vi "parse_to_rio.vi"(4 "error in":errorcluster, 7 "msg in":string) -> (0 "error out":errorcluster, 2 "to_rio":cluster{"set_speed":dbl, "set_steering":dbl}, 3 "msg out":string)   [LabVIEW 2016]
uses:
  <userlib>/ROS for LabVIEW Software/ROS/MessageParsing/std_msgs/subs/parse_float64_scalar.vi
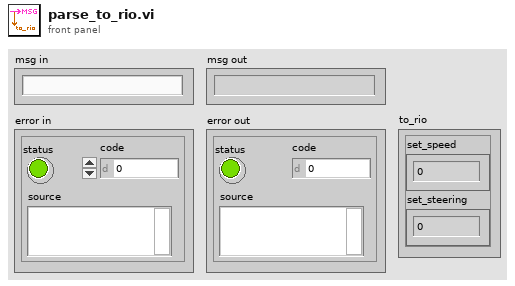
[diagram p1: front panel]
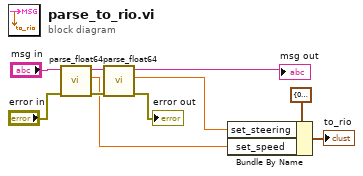
[diagram p0: block diagram]
diagram:
  n1 = call-poly <userlib>:"parse_float64.vi"("error in"="error in", "msg in"="msg in") -> ("error out"=w4:errorcluster, "number"=w1:dbl, "msg out"=w3:string)  [unwired: 3 in]
  n2 = call-poly <userlib>:"parse_float64.vi"("error in"=w4, "msg in"=w3) -> ("error out"=→"error out":errorcluster, "number"=w2:dbl, "msg out"=→"msg out":string)  [unwired: 3 in]
  n3 = Bundle By Name(cluster=cluster{"set_speed":dbl, "set_steering":dbl} {"set_speed"=0.0, "set_steering"=0.0}, "set_steering"=w2, "set_speed"=w1) -> (→"to_rio":cluster{"set_speed":dbl, "set_steering":dbl})
